vi "Interpolate.vi"(8 "Angles":dbl[](array[numeric]), 9 "DesiredAngle":dbl, 10 "Values":dbl[](array[numeric]), 11 "Indexes":dbl[](array[numeric])) -> (3 "InterpolatedValue":dbl)   [LabVIEW 2012, in "LinearInterpolation.lvclass"]
uses:
  LinearInterpolation.lvclass
  <vilib>/Analysis/NI_AALPro.lvlib
panel:
  out "X Values":dbl[](array[numeric])
  out "x > y? 2":bool
  in  "Angles 2":dbl[](array[numeric])
  out "Indexes 3":dbl[](array[numeric])
  out "InterpolatedValue 2":dbl
  in  "DesiredAngle 2":dbl
  in  "Values 2":void[](array[numeric])
  in  "Indexes 4":dbl[](array[numeric])
  out "Indexes 2":dbl[](array[numeric])
  out "Y values":dbl[](array[numeric])
  out "x = y?":bool
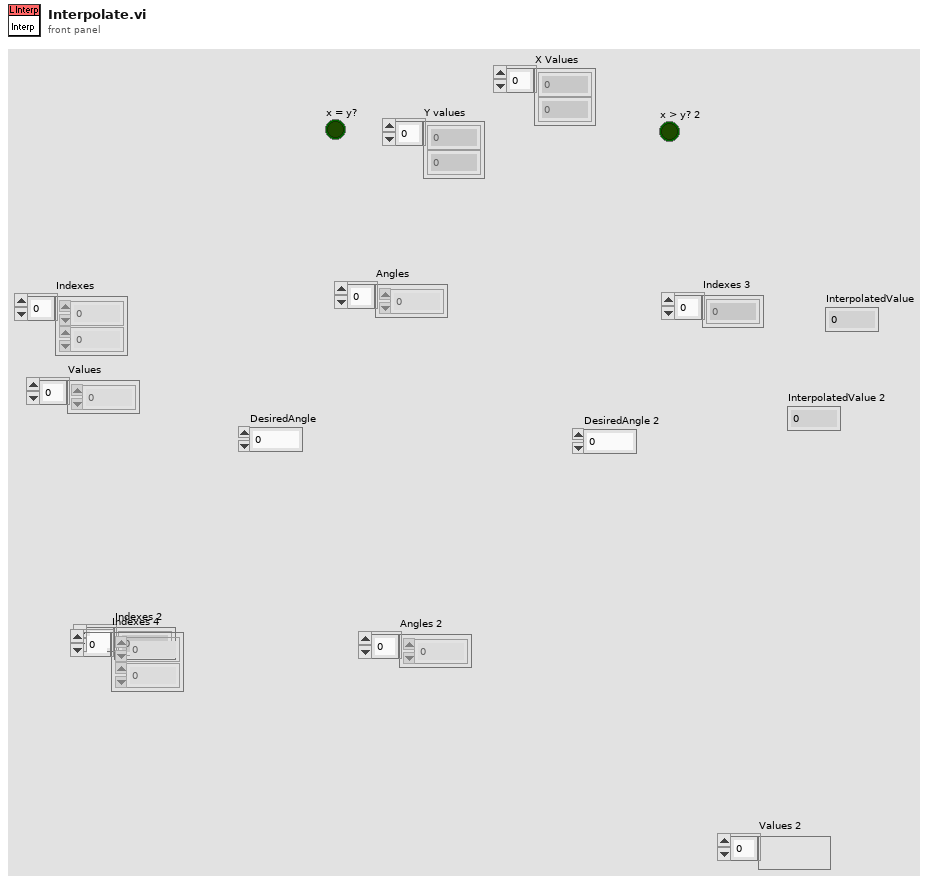
[diagram p1: front panel]
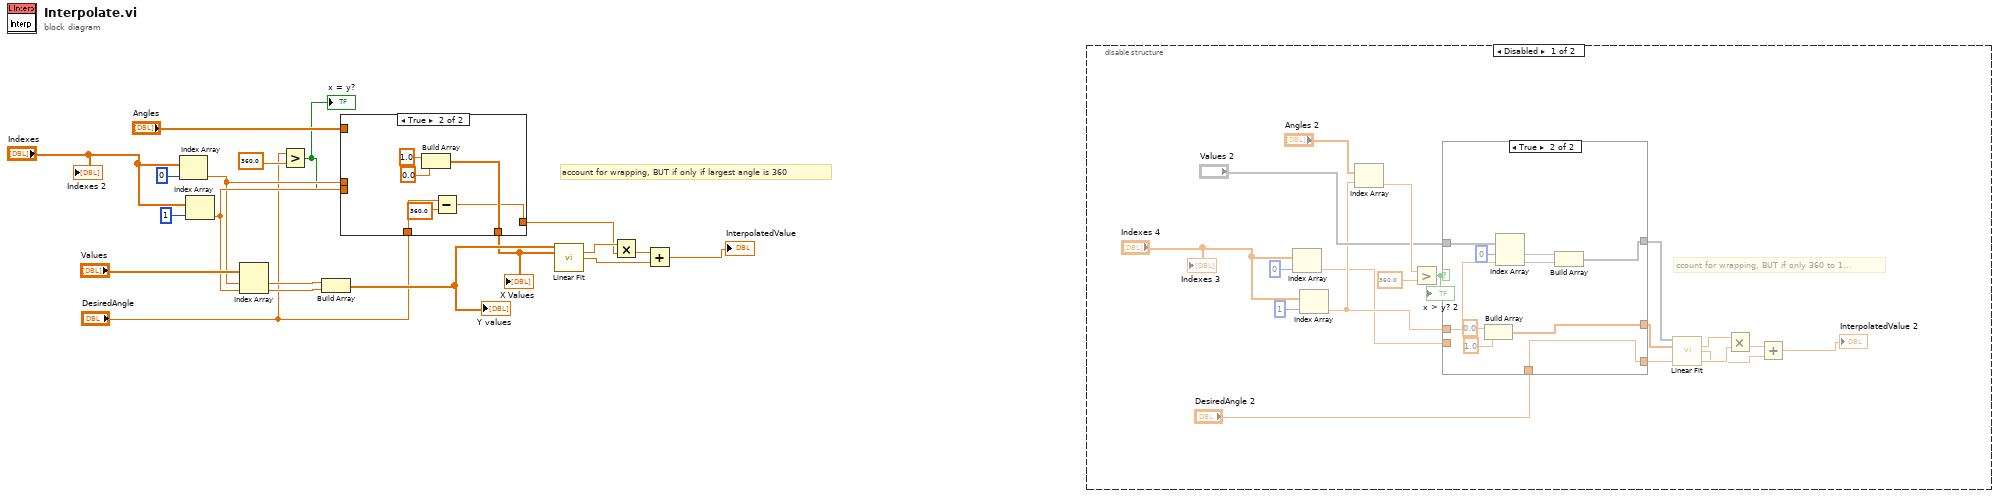
[diagram p0: block diagram]
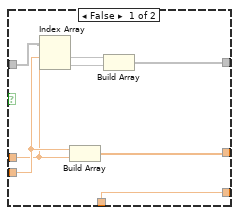
[diagram p2: hidden frame]
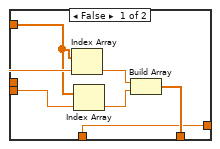
[diagram p4: hidden frame]
diagram:
  # "account for wrapping, BUT if only if largest angle is 360"
  n1 = Index Array(array="Indexes", index=0) -> (element=w6:dbl)
  n2 = Index Array(array="Indexes", index=1) -> (element=w7:dbl)
  n3 = Index Array(array="Values", index #1=w6, index #2=w7) -> (element #1=w5:dbl, element #2=w4:dbl)
  n4 = Greater?(x="DesiredAngle", y=360.0 ("x")) -> (0:w2:bool)
  "x = y?" <- w2
  n5 = Build Array(w5, w4) -> (w19:dbl[])
  "Y values" <- w19
  n6 = case shown="True" w2 {
    tunnel: w7 -> [w21 _]
    tunnel: [w26 w30] -> w9
    tunnel: w6 -> [w24 _]
    tunnel: "DesiredAngle" -> [w25 w29]
    tunnel: [w25 w27] -> w10
    tunnel: "Angles" -> [w20 _]
    frame False {
      n7 = Index Array(array=w20, index=w24) -> (element=w22:dbl)
      n8 = Index Array(array=w20, index=w21) -> (element=w23:dbl)
      n9 = Build Array(w22, w23) -> (w26:dbl[])
    }
    frame True {
      n10 = Build Array(1.0 ("element"), 0.0 ("element")) -> (w30:dbl[])
      n11 = Subtract(x=w29, y=360.0) -> (x-y=w27:dbl)
    }
  }
  "X Values" <- w9
  n12 = call <vilib>:"Linear Fit.vi"("Y"=w19, "X"=w9) -> ("slope"=w18:dbl, "intercept"=w16:dbl)  [unwired: 9 in, 3 out]
  n13 = Multiply(x=w18, y=w10) -> (x*y=w17:dbl)
  n14 = Add(x=w17, y=w16) -> (x+y=→"InterpolatedValue":dbl)
  n15 = disable-structure shown="Disabled" {
    frame Disabled {
      # "ccount for wrapping, BUT if only 360 to 1..."
      n16 = Index Array(array="Indexes 4", index=0) -> (element=w41:dbl)
      n17 = Index Array(array="Indexes 4", index=1) -> (element=w46:dbl)
      n18 = Index Array(array="Angles 2", index=w46) -> (element=w49:dbl)
      n19 = Greater?(x=w49, y=360.0) -> (0:w42:bool)
      "x > y? 2" <- w42
      n20 = case shown="True" w42 {
        tunnel: w46 -> [w55 w60]
        tunnel: [w58 w66] -> w38
        tunnel: w41 -> [w56 _]
        tunnel: "DesiredAngle 2" -> [w57 w65]
        tunnel: [w57 w65] -> w44
        tunnel: [w52 w61] -> w45
        tunnel: "Values 2" -> [w51 w62]
        frame False {
          n21 = Index Array(array=w51, index #1=w56, index #2=w55) -> (element #1=w54, element #2=w53)
          n22 = Build Array(w56, w55) -> (w58:dbl[])
          n23 = Build Array(w54, w53) -> (w52:void[])
        }
        frame True {
          n24 = Build Array(0.0 ("element"), 1.0 ("element")) -> (w66:dbl[])
          n25 = Index Array(array=w62, index #1=0 ("index"), index #2=w60) -> (element #1=w63, element #2=w64)
          n26 = Build Array(w63, w64) -> (w61:void[])
        }
      }
      n27 = call <vilib>:"Linear Fit.vi"("Y"=w45, "X"=w38) -> ("slope"=w33:dbl, "intercept"=w35:dbl)  [unwired: 9 in, 3 out]
      n28 = Multiply(x=w33, y=w44) -> (x*y=w34:dbl)
      n29 = Add(x=w34, y=w35) -> (x+y=→"InterpolatedValue 2":dbl)
      "Indexes 3" <- "Indexes 4"
    }
    frame Enabled {
    }
  }
  "Indexes 2" <- "Indexes"
